vi "query database for schedules.vi"() -> ()   [LabVIEW 2015]
uses:
  Choose Schedule.ctl
  <vilib>/addons/database/Connection.llb/DB Tools Open Connec (Path).vi
  <vilib>/addons/database/NI_Database_API.lvlib
panel:
  out "Numeric 3":i32
  out "String":string
  out "subarray":string[][](array[string])
  out "Numeric 2":i32
  out "Numeric":i32
  out "output array":string[](array[string])
  out "error out":errorcluster
  out "output cluster":T1
  in  "Array Schedule":T1[](array[typedef])
  out "data 2":string[][](array[string])
  out "data":variant[][](array[variant])
  # "ID               Name                       Step            Gas          Time"
  # "ID               Name                       Step            Gas          Time"
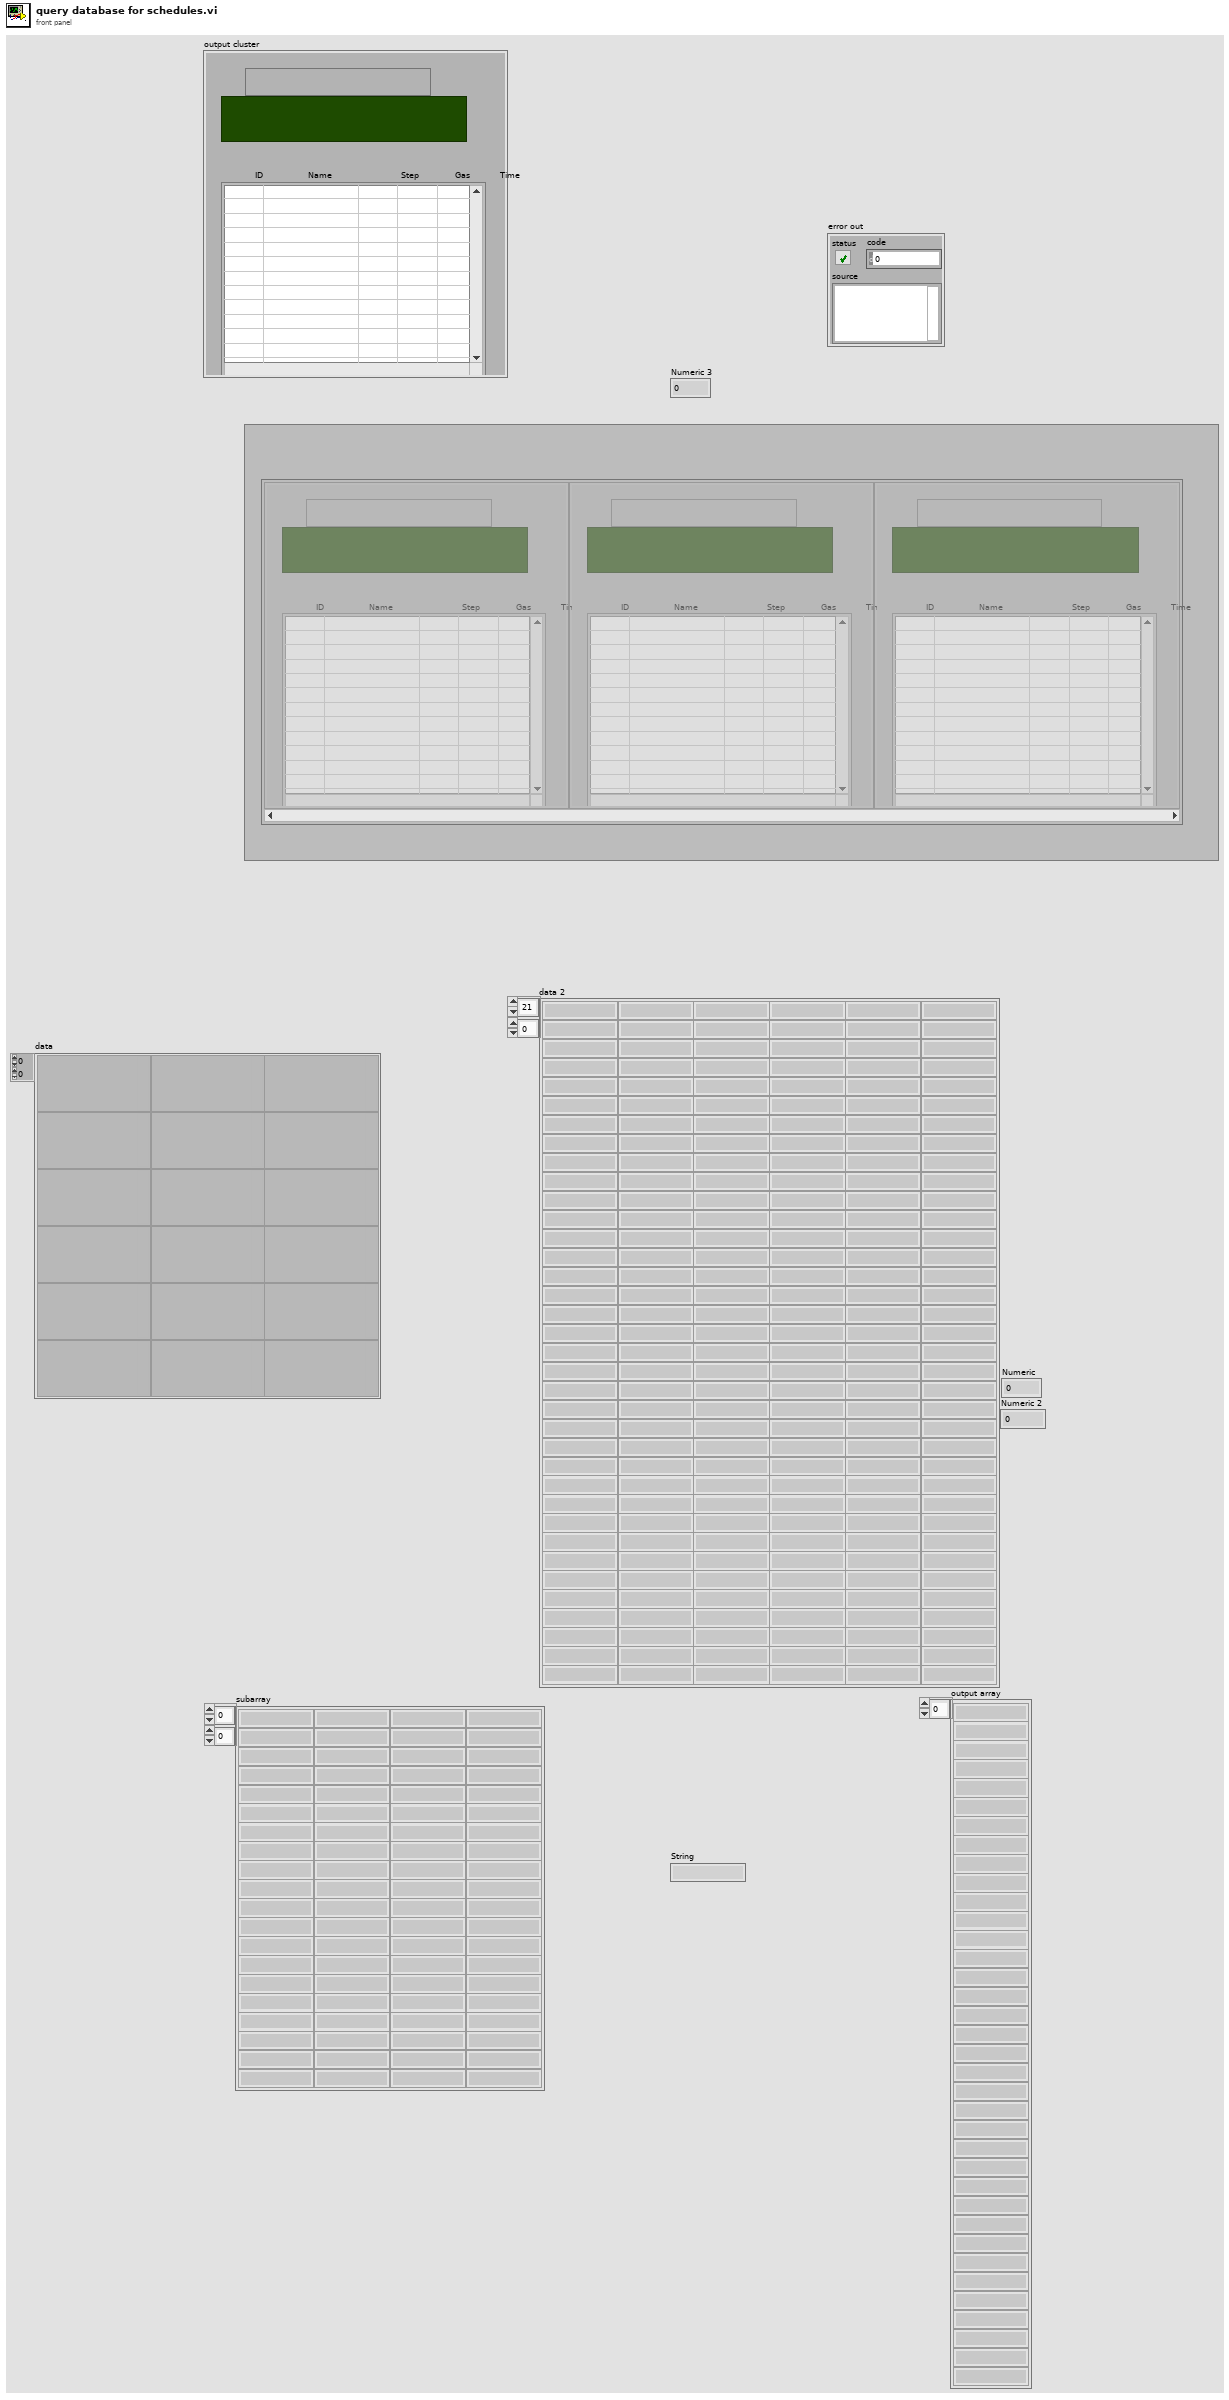
[diagram p1: front panel]
types:
  T1 = typedef "Choose Schedule.ctl" = cluster{"Schedule Table":string[][], "Boolean":bool, "Schedule Name":string}
  T2 = typedef "NI_Database_API.lvlib/Conn ObjectReference.ctl" = refnum<k1>
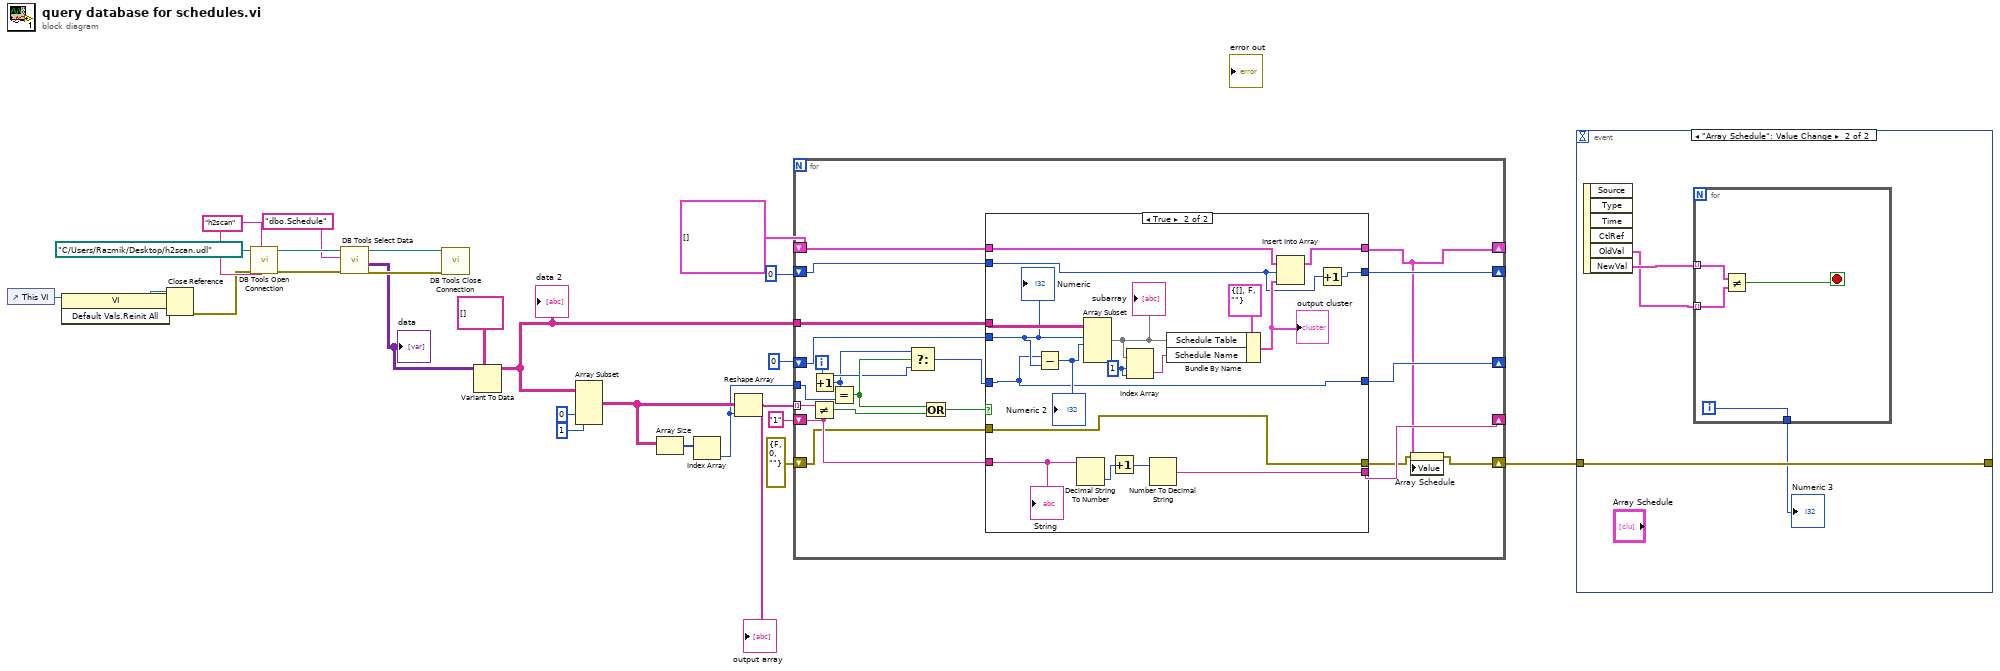
[diagram p0: block diagram]
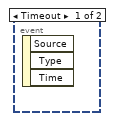
[diagram p2: hidden frame]
diagram:
  w25 = "h2scan" ("userID")
  n1 = control-ref of="This VI"() -> (w6:refnum<vi>)
  n2 = invoke class="VI" method="Default Vals.Reinit All"(reference=w6) -> (reference out=w7:refnum<vi>, error out=w8:errorcluster)  [unwired: 2 in, 1 out]
  n3 = Close Reference(reference=w7, error in (no error)=w8) -> (error out=w5:errorcluster)
  n4 = call-poly <vilib>:"DB Tools Open Connection.vi"("password"=w25, "userID"=w25, "error in (no error)"=w5, "connection information"=path "C:/Users/Razmik/Desktop/h2scan.udl") -> ("error out"=w23:errorcluster, "connection reference"=w24:T2)  [unwired: 4 in]
  n5 = call <vilib>:"DB Tools Select Data.vi"("error in (no error)"=w23, "table"="dbo.Schedule", "connection reference"=w24) -> ("error out"=w20:errorcluster, "data"=w19:variant[][], "connection reference out"=w21:T2)  [unwired: 3 in]
  "data" <- w19
  n6 = call <vilib>:"DB Tools Close Connection.vi"("error in (no error)"=w20, "connection reference"=w21) -> ()  [unwired: 5 in, 1 out]
  n7 = Variant To Data(type=string[][] [], Variant=w19) -> (data=w11:string[][])  [unwired: 1 in, 1 out]
  "data 2" <- w11
  n8 = Array Subset(array=w11, index (col)=0 ("index"), length (col)=1 ("length")) -> (w15:string[][])  [unwired: 2 in]
  n9 = Array Size(array=w15) -> (size(s)=w14:i32[])
  n10 = Index Array(array=w14) -> (element=w2:i32)  [unwired: 1 in]
  n11 = Reshape Array(w15, w2) -> (w13:string[])
  "output array" <- w13
  n12 = for {
    tunnel: w13 -> [w46] mode=indexing
    shift-right: [w37] -> _
    shift-left: "1" -> [w45]
    tunnel: w11 -> [w43]
    shift-right: [w41] -> _
    shift-left: 0 -> [w42]
    shift-right: [w27] -> w1
    shift-left: errorcluster {"status"=FALSE, "code"=0, "source"=""} ("error out") -> [w40]
    shift-right: [w29] -> _
    shift-left: T1[] [] -> [w44]
    shift-right: [w38] -> _
    shift-left: 0 -> [w39]
    tunnel: w2 -> [w36]
    i -> [w32]
    n13 = Not Equal?(x=w46, y=w45) -> (x != y?=w35:bool)
    n14 = Increment(x=w32) -> (x+1=w31:i32)
    n15 = Equal?(x=w31, y=w36) -> (x = y?=w33:bool)
    n16 = Select(t=w31, s=w33, f=w32) -> (s? t:f=w30:i32)
    n17 = Or(x=w33, y=w35) -> (x .or. y?=w34:bool)
    n18 = case shown="True" w34 {
      tunnel: w45 -> [w51 w69]
      tunnel: [w51 w67] -> w37
      tunnel: w44 -> [w48 w61]
      tunnel: w43 -> [_ w66]
      tunnel: w42 -> [w50 w57]
      tunnel: w30 -> [_ w55]
      tunnel: [w50 w55] -> w41
      tunnel: [w49 w58] -> w28
      tunnel: w40 -> [w49 w58]
      tunnel: [w48 w60] -> w29
      tunnel: w39 -> [w47 w54]
      tunnel: [w47 w53] -> w38
      frame False {
      }
      frame True {
        w63 = 1 ("index (row)")
        n19 = Subtract(x=w55, y=w57) -> (x-y=w56:i32)
        "Numeric 2" <- w56
        n20 = Decimal String To Number(string=w69) -> (number=w52:i32)  [unwired: 2 in, 1 out]
        n21 = Array Subset(array=w66, index (row)=w57, length (row)=w56) -> (w64:string[][])  [unwired: 2 in]
        "subarray" <- w64
        n22 = Increment(x=w52) -> (x+1=w68:i32)
        n23 = Index Array(array=w64, index (row)=w63, index (col)=w63) -> (element=w59:string)
        n24 = Number To Decimal String(number=w68) -> (decimal integer string=w67:string)  [unwired: 1 in]
        n25 = Bundle By Name(cluster=T1 {"Schedule Table"=[], "Boolean"=FALSE, "Schedule Name"=""} ("Schedule"), "Schedule Table"=w64, "Schedule Name"=w59) -> (w62:T1)
        "output cluster" <- w62
        n26 = Insert Into Array(array=w61, index=w54, new element=w62) -> (w60:T1[])
        n27 = Increment(x=w54) -> (x+1=w53:i32)
        "Numeric" <- w57
        "String" <- w69
      }
    }
    n28 = property on="Array Schedule" class="Arr"(error in=w28, "Value"=w29) -> (error out=w27:errorcluster)  [unwired: 1 in, 1 out]
  }
  n29 = event shown="[1] \"Array Schedule\": Value Change" {
    selector: _ -> [_ _]
    dyn-events: _ -> [_ _]
    timeout: _ -> [_ _]
    tunnel: w1 -> [_ w71]
    tunnel: [_ w71] -> _
    event Timeout {
      n30 = event-data() -> ()  [unwired: 1 in, 3 out]
    }
    event "Array Schedule": Value Change {
      n31 = event-data() -> ("OldVal"=w72:T1[], "NewVal"=w73:T1[])  [unwired: 1 in, 4 out]
      n32 = for {
        tunnel: w73 -> [w77] mode=indexing
        tunnel: w72 -> [w76] mode=indexing
        tunnel: [w74] -> w70
        i -> [w74]
        stop <- w75 stop-if-true
        n33 = Not Equal?(x=w77, y=w76) -> (x != y?=w75:bool)
      }
      "Numeric 3" <- w70
    }
  }
